vi "Create Webform.vi"(6 "Under Construction":bool[](array[boolean]), 8 "error in (no error)":errorcluster, 9 "Mathcad version":i32, 10 "Method Name":string, 11 "Method":T2) -> (0 "error out":errorcluster, 3 "HTML string":string)   [LabVIEW 2012, in "Design Server.lvlib"]
uses:
  Design Server.lvlib
  Method.ctl
  RequestKeys.ctl
  Folders.ctl
  <vilib>/Utility/file.llb/Read From Spreadsheet File (string).vi
panel:
  in  "Required":bool[](array[boolean])=[TRUE, TRUE, TRUE, TRUE, FALSE, FALSE, FALSE, FALSE]
  out "String":string
  in  "Load countries":bool
  in  "Country codes":string[][](array[string])=[["\"Table 1. Countries, Dependencies, and Areas of Special Sovereignty (Alphabetical by Name)\"", "", ""], ["http://earth-info.nga.mil/gns/html/gazetteers2.html", "", ""], ["Code", "Name (Upper Case)", "Name (Upper and Lower Case)"], ["AF", "AFGHANISTAN", "Afghanistan"], ["AX", "AKROTIRI", "Akrotiri"], ["AL", "ALBANIA", "Albania"], ["AG", "ALGERIA", "Algeria"], ["AQ", "AMERICAN SAMOA", "American Samoa"], ["AN", "ANDORRA", "Andorra"], ["AO", "ANGOLA", "Angola"], ["AV", "ANGUILLA", "Anguilla"], ["AY", "ANTARCTICA", "Antarctica"], ["AC", "ANTIGUA AND BARBUDA", "Antigua and Barbuda"], ["AR", "ARGENTINA", "Argentina"], ["AM", "ARMENIA", "Armenia"], ["AA", "ARUBA", "Aruba"], ["AT", "ASHMORE AND CARTIER ISLANDS", "Ashmore and Cartier Islands"], ["AS", "AUSTRALIA", "Australia"], ["AU", "AUSTRIA", "Austria"], ["AJ", "AZERBAIJAN", "Azerbaijan"], ["BF", "BAHAMAS, THE", "Bahamas, The"], ["BA", "BAHRAIN", "Bahrain"], ["FQ", "BAKER ISLAND", "Baker Island"], ["BG", "BANGLADESH", "Bangladesh"], ["BB", "BARBADOS", "Barbados"], ["BS", "BASSAS DA INDIA", "Bassas da India"], ["BO", "BELARUS", "Belarus"], ["BE", "BELGIUM", "Belgium"], ["BH", "BELIZE", "Belize"], ["BN", "BENIN", "Benin"], ["BD", "BERMUDA", "Bermuda"], ["BT", "BHUTAN", "Bhutan"], ["BL", "BOLIVIA", "Bolivia"], ["BK", "BOSNIA AND HERZEGOVINA", "Bosnia and Herzegovina"], ["BC", "BOTSWANA", "Botswana"], ["BV", "BOUVET ISLAND", "Bouvet Island"], ["BR", "BRAZIL", "Brazil"], ["IO", "BRITISH INDIAN OCEAN TERRITORY", "British Indian Ocean Territory"], ["BX", "BRUNEI", "Brunei"], ["BU", "BULGARIA", "Bulgaria"], ["UV", "BURKINA FASO", "Burkina Faso"], ["BM", "BURMA", "Burma"], ["BY", "BURUNDI", "Burundi"], ["CB", "CAMBODIA", "Cambodia"], ["CM", "CAMEROON", "Cameroon"], ["CA", "CANADA", "Canada"], ["CV", "CAPE VERDE", "Cape Verde"], ["CJ", "CAYMAN ISLANDS", "Cayman Islands"], ["CT", "CENTRAL AFRICAN REPUBLIC", "Central African Republic"], ["CD", "CHAD", "Chad"], ["CI", "CHILE", "Chile"], ["CH", "CHINA", "China"], ["KT", "CHRISTMAS ISLAND", "Christmas Island"], ["IP", "CLIPPERTON ISLAND", "Clipperton Island"], ["CK", "COCOS (KEELING) ISLANDS", "Cocos (Keeling) Islands"], ["CO", "COLOMBIA", "Colombia"], ["CN", "COMOROS", "Comoros"], ["CF", "CONGO (BRAZZAVILLE)", "Congo (Brazzaville)"], ["CG", "CONGO (KINSHASA)", "Congo (Kinshasa)"], ["CW", "COOK ISLANDS", "Cook Islands"], ["CR", "CORAL SEA ISLANDS", "Coral Sea Islands"], ["CS", "COSTA RICA", "Costa Rica"], ["IV", "CÔTE D’IVOIRE", "Côte d’Ivoire"], ["HR", "CROATIA", "Croatia"], ["CU", "CUBA", "Cuba"], ["UC", "CURAÇAO", "Curaçao"], ["CY", "CYPRUS", "Cyprus"], ["EZ", "CZECH REPUBLIC", "Czech Republic"], ["DA", "DENMARK", "Denmark"], ["DX", "DHEKELIA", "Dhekelia"], ["DJ", "DJIBOUTI", "Djibouti"], ["DO", "DOMINICA", "Dominica"], ["DR", "DOMINICAN REPUBLIC", "Dominican Republic"], ["EC", "ECUADOR", "Ecuador"], ["EG", "EGYPT", "Egypt"], ["ES", "EL SALVADOR", "El Salvador"], ["EK", "EQUATORIAL GUINEA", "Equatorial Guinea"], ["ER", "ERITREA", "Eritrea"], ["EN", "ESTONIA", "Estonia"], ["ET", "ETHIOPIA", "Ethiopia"], ["PJ", "ETOROFU, HABOMAI, KUNASHIRI, AND SHIKOTAN ISLANDS", "Etorofu, Habomai, Kunashiri, and Shikotan Islands"], ["EU", "EUROPA ISLAND", "Europa Island"], ["FK", "FALKLAND ISLANDS (ISLAS MALVINAS)", "Falkland Islands (Islas Malvinas)"], ["FO", "FAROE ISLANDS", "Faroe Islands"], ["FJ", "FIJI", "Fiji"], ["FI", "FINLAND", "Finland"], ["FR", "FRANCE", "France"], ["FG", "FRENCH GUIANA", "French Guiana"], ["FP", "FRENCH POLYNESIA", "French Polynesia"], ["FS", "FRENCH SOUTHERN AND ANTARCTIC LANDS", "French Southern and Antarctic Lands"], ["GB", "GABON", "Gabon"], ["GA", "GAMBIA, THE", "Gambia, The"], ["GZ", "GAZA STRIP", "Gaza Strip"], ["GG", "GEORGIA", "Georgia"], ["GM", "GERMANY", "Germany"], ["GH", "GHANA", "Ghana"], ["GI", "GIBRALTAR", "Gibraltar"], ["GO", "GLORIOSO ISLANDS", "Glorioso Islands"], ["GR", "GREECE", "Greece"], ["GL", "GREENLAND", "Greenland"], ["GJ", "GRENADA", "Grenada"], ["GP", "GUADELOUPE", "Guadeloupe"], ["GQ", "GUAM", "Guam"], ["GT", "GUATEMALA", "Guatemala"], ["GK", "GUERNSEY", "Guernsey"], ["GV", "GUINEA", "Guinea"], ["PU", "GUINEA-BISSAU", "Guinea-Bissau"], ["GY", "GUYANA", "Guyana"], ["HA", "HAITI", "Haiti"], ["HM", "HEARD ISLAND AND MCDONALD  ISLANDS", "Heard Island and McDonald  Islands"], ["HO", "HONDURAS", "Honduras"], ["HK", "HONG KONG", "Hong Kong"], ["HQ ", "HOWLAND ISLAND", "Howland Island"], ["HU", "HUNGARY", "Hungary"], ["IC", "ICELAND", "Iceland"], ["IN", "INDIA", "India"], ["ID", "INDONESIA", "Indonesia"], ["IR", "IRAN", "Iran"], ["IZ", "IRAQ", "Iraq"], ["EI", "IRELAND", "Ireland"], ["IM", "ISLE OF MAN", "Isle of Man"], ["IS", "ISRAEL", "Israel"], ["IT", "ITALY", "Italy"], ["JM", "JAMAICA", "Jamaica"], ["JN", "JAN MAYEN", "Jan Mayen"], ["JA", "JAPAN", "Japan"], ["DQ", "JARVIS ISLAND", "Jarvis Island"], ["JE", "JERSEY", "Jersey"], ["JQ", "JOHNSTON ATOLL", "Johnston Atoll"], ["JO", "JORDAN", "Jordan"], ["JU", "JUAN DE NOVA ISLAND", "Juan de Nova Island"], ["KZ", "KAZAKHSTAN", "Kazakhstan"], ["KE", "KENYA", "Kenya"], ["KQ", "KINGMAN REEF", "Kingman Reef"], ["KR", "KIRIBATI", "Kiribati"], ["KN", "KOREA, NORTH", "Korea, North"], ["KS", "KOREA, SOUTH", "Korea, South"], ["KV", "KOSOVO", "Kosovo"], ["KU", "KUWAIT", "Kuwait"], ["KG", "KYRGYZSTAN", "Kyrgyzstan"], ["LA", "LAOS", "Laos"], ["LG", "LATVIA", "Latvia"], ["LE", "LEBANON", "Lebanon"], ["LT", "LESOTHO", "Lesotho"], ["LI", "LIBERIA", "Liberia"], ["LY", "LIBYA", "Libya"], ["LS", "LIECHTENSTEIN", "Liechtenstein"], ["LH", "LITHUANIA", "Lithuania"], ["LU", "LUXEMBOURG", "Luxembourg"], ["MC", "MACAU", "Macau"], ["MK", "MACEDONIA", "Macedonia"], ["MA", "MADAGASCAR", "Madagascar"], ["MI", "MALAWI", "Malawi"], ["MY", "MALAYSIA", "Malaysia"], ["MV", "MALDIVES", "Maldives"], ["ML", "MALI", "Mali"], ["MT", "MALTA", "Malta"], ["RM", "MARSHALL ISLANDS", "Marshall Islands"], ["MB", "MARTINIQUE", "Martinique"], ["MR", "MAURITANIA", "Mauritania"], ["MP", "MAURITIUS", "Mauritius"], ["MF", "MAYOTTE", "Mayotte"], ["MX", "MEXICO", "Mexico"], ["FM", "MICRONESIA, FEDERATED STATES OF", "Micronesia, Federated States of"], ["MQ ", "MIDWAY ISLANDS", "Midway Islands"], ["MD", "MOLDOVA", "Moldova"], ["MN", "MONACO", "Monaco"], ["MG", "MONGOLIA", "Mongolia"], ["MJ", "MONTENEGRO", "Montenegro"], ["MH", "MONTSERRAT", "Montserrat"], ["MO", "MOROCCO", "Morocco"], ["MZ", "MOZAMBIQUE", "Mozambique"], ["WA", "NAMIBIA", "Namibia"], ["NR", "NAURU", "Nauru"], ["BQ", "NAVASSA ISLAND", "Navassa Island"], ["NP", "NEPAL", "Nepal"], ["NL", "NETHERLANDS", "Netherlands"], ["NC", "NEW CALEDONIA", "New Caledonia"], ["NZ", "NEW ZEALAND", "New Zealand"], ["NU", "NICARAGUA", "Nicaragua"], ["NG", "NIGER", "Niger"], ["NI", "NIGERIA", "Nigeria"], ["NE", "NIUE", "Niue"], ["NF", "NORFOLK ISLAND", "Norfolk Island"], ["CQ", "NORTHERN MARIANA ISLANDS", "Northern Mariana Islands"], ["NO", "NORWAY", "Norway"], ["MU", "OMAN", "Oman"], ["PK", "PAKISTAN", "Pakistan"], ["PS", "PALAU", "Palau"], ["LQ", "PALMYRA ATOLL", "Palmyra Atoll"], ["PM", "PANAMA", "Panama"], ["PP", "PAPUA NEW GUINEA", "Papua New Guinea"], ["PF", "PARACEL ISLANDS", "Paracel Islands"], ["PA", "PARAGUAY", "Paraguay"], ["PE", "PERU", "Peru"], ["RP", "PHILIPPINES", "Philippines"], ["PC", "PITCAIRN ISLANDS", "Pitcairn Islands"], ["PL", "POLAND", "Poland"], ["PO", "PORTUGAL", "Portugal"], ["RQ", "PUERTO RICO", "Puerto Rico"], ["QA", "QATAR", "Qatar"], ["RE", "REUNION", "Reunion"], ["RO", "ROMANIA", "Romania"], ["RS", "RUSSIA", "Russia"], ["RW", "RWANDA", "Rwanda"], ["TB", "SAINT BARTHELEMY", "Saint Barthelemy"], ["SH", "SAINT HELENA, ASCENSION, AND TRISTAN DA CUNHA", "Saint Helena, Ascension, and Tristan da Cunha"], ["SC", "SAINT KITTS AND NEVIS", "Saint Kitts and Nevis"], ["ST", "SAINT LUCIA", "Saint Lucia"], ["RN", "SAINT MARTIN", "Saint Martin"], ["SB", "SAINT PIERRE AND MIQUELON", "Saint Pierre and Miquelon"], ["VC", "SAINT VINCENT AND THE GRENADINES", "Saint Vincent and the Grenadines"], ["WS", "SAMOA", "Samoa"], ["SM", "SAN MARINO", "San Marino"], ["TP", "SAO TOME AND PRINCIPE", "Sao Tome and Principe"], ["SA", "SAUDI ARABIA", "Saudi Arabia"], ["SG", "SENEGAL", "Senegal"], ["RI", "SERBIA", "Serbia"], ["SE", "SEYCHELLES", "Seychelles"], ["SL", "SIERRA LEONE", "Sierra Leone"], ["SN", "SINGAPORE", "Singapore"], ["NN", "SINT MAARTEN", "Sint Maarten"], ["LO", "SLOVAKIA", "Slovakia"], ["SI", "SLOVENIA", "Slovenia"], ["BP", "SOLOMON ISLANDS", "Solomon Islands"], ["SO", "SOMALIA", "Somalia"], ["SF", "SOUTH AFRICA", "South Africa"], ["SX", "SOUTH GEORGIA AND SOUTH SANDWICH ISLANDS", "South Georgia and South Sandwich Islands"], ["OD", "SOUTH SUDAN", "South Sudan"], ["SP", "SPAIN", "Spain"], ["PG", "SPRATLY ISLANDS", "Spratly Islands"], ["CE", "SRI LANKA", "Sri Lanka"], ["SU", "SUDAN", "Sudan"], ["NS", "SURINAME", "Suriname"], ["SV", "SVALBARD", "Svalbard"], ["WZ", "SWAZILAND", "Swaziland"], ["SW", "SWEDEN", "Sweden"], ["SZ", "SWITZERLAND", "Switzerland"], ["SY", "SYRIA", "Syria"], ["TW", "TAIWAN", "Taiwan"], ["TI", "TAJIKISTAN", "Tajikistan"], ["TZ", "TANZANIA", "Tanzania"], ["TH", "THAILAND", "Thailand"], ["TT", "TIMOR-LESTE", "Timor-Leste"], ["TO", "TOGO", "Togo"], ["TL", "TOKELAU", "Tokelau"], ["TN", "TONGA", "Tonga"], ["TD", "TRINIDAD AND TOBAGO", "Trinidad and Tobago"], ["TE", "TROMELIN ISLAND", "Tromelin Island"], ["TS", "TUNISIA", "Tunisia"], ["TU", "TURKEY", "Turkey"], ["TX", "TURKMENISTAN", "Turkmenistan"], ["TK", "TURKS AND CAICOS ISLANDS", "Turks and Caicos Islands"], ["TV", "TUVALU", "Tuvalu"], ["UG", "UGANDA", "Uganda"], ["UP", "UKRAINE", "Ukraine"], ["AE", "UNITED ARAB EMIRATES", "United Arab Emirates"], ["UK", "UNITED KINGDOM", "United Kingdom"], ["US", "UNITED STATES", "United States"], ["UY", "URUGUAY", "Uruguay"], ["UZ", "UZBEKISTAN", "Uzbekistan"], ["NH", "VANUATU", "Vanuatu"], ["VT", "VATICAN CITY", "Vatican City"], ["VE", "VENEZUELA", "Venezuela"], ["VM", "VIETNAM", "Vietnam"], ["VI", "VIRGIN ISLANDS, BRITISH", "Virgin Islands, British"], ["VQ ", "VIRGIN ISLANDS, U.S.", "Virgin Islands, U.S."], ["WQ", "WAKE ISLAND", "Wake Island"], ["WF", "WALLIS AND FUTUNA", "Wallis and Futuna"], ["WE", "WEST BANK", "West Bank"], ["WI", "WESTERN SAHARA", "Western Sahara"], ["YM", "YEMEN", "Yemen"], ["ZA", "ZAMBIA", "Zambia"], ["ZI", "ZIMBABWE", "Zimbabwe"]]
  in  "Path":path=path "C:/Users/design/Documents/LabVIEW Code/AguaClara Design Server/Country codes.txt"
  in  "Request Keys":T1=enum."ProjectNotes"
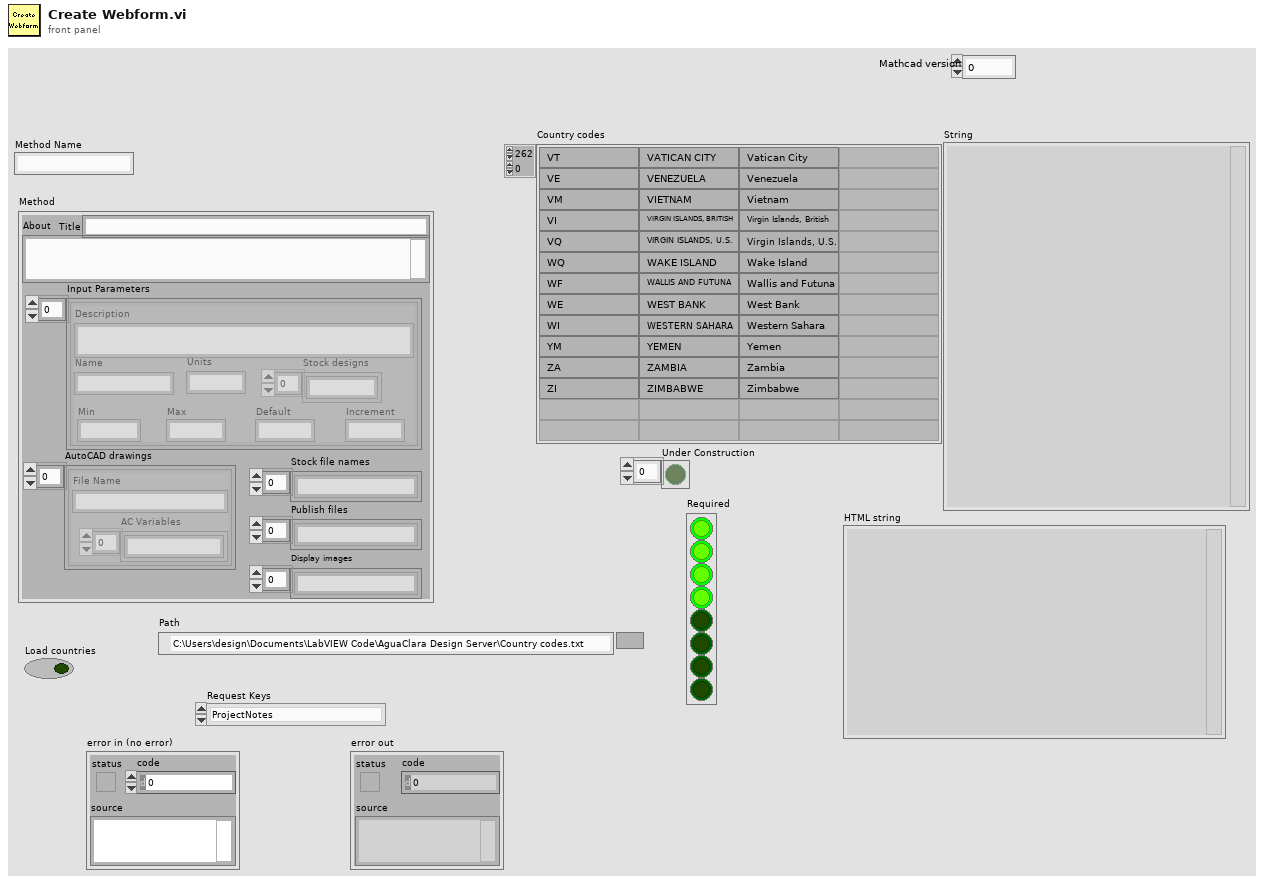
[diagram p1: front panel]
types:
  T1 = typedef "Design Server.lvlib/RequestKeys.ctl" = enum16{"FormName", "Name", "Email", "Organization", "Country", "ProjectTitle", "ProjectCity", "ProjectState", "ProjectNotes"}
  T2 = typedef "Method.ctl" = cluster{"Title":string, "About":string, "Input Parameters":cluster{"Description":string, "Name":string, "Min":string, "Max":string, "Default":string, "Units":string, "Increment":string, "Stock designs":string[]}[], "AutoCAD drawings":cluster{"File Name":string, "AC Variables":string[]}[], "Stock file names":string[], "Publish files":string[], "Display images":string[]}
  T3 = typedef "Design Server.lvlib/Folders.ctl" = enum16{"MathcadMethods", "RequestedDesigns", "CompletedDesigns", "MathcadCode", "CollabnetSVN.exe"}
  T4 = enum16{"open", "replace", "create", "open or create", "replace or create", "replace or create with confirmation"}
  T5 = cluster{"Description":string, "Name":string, "Min":string, "Max":string, "Default":string, "Units":string, "Increment":string, "Stock designs":string[]}[]
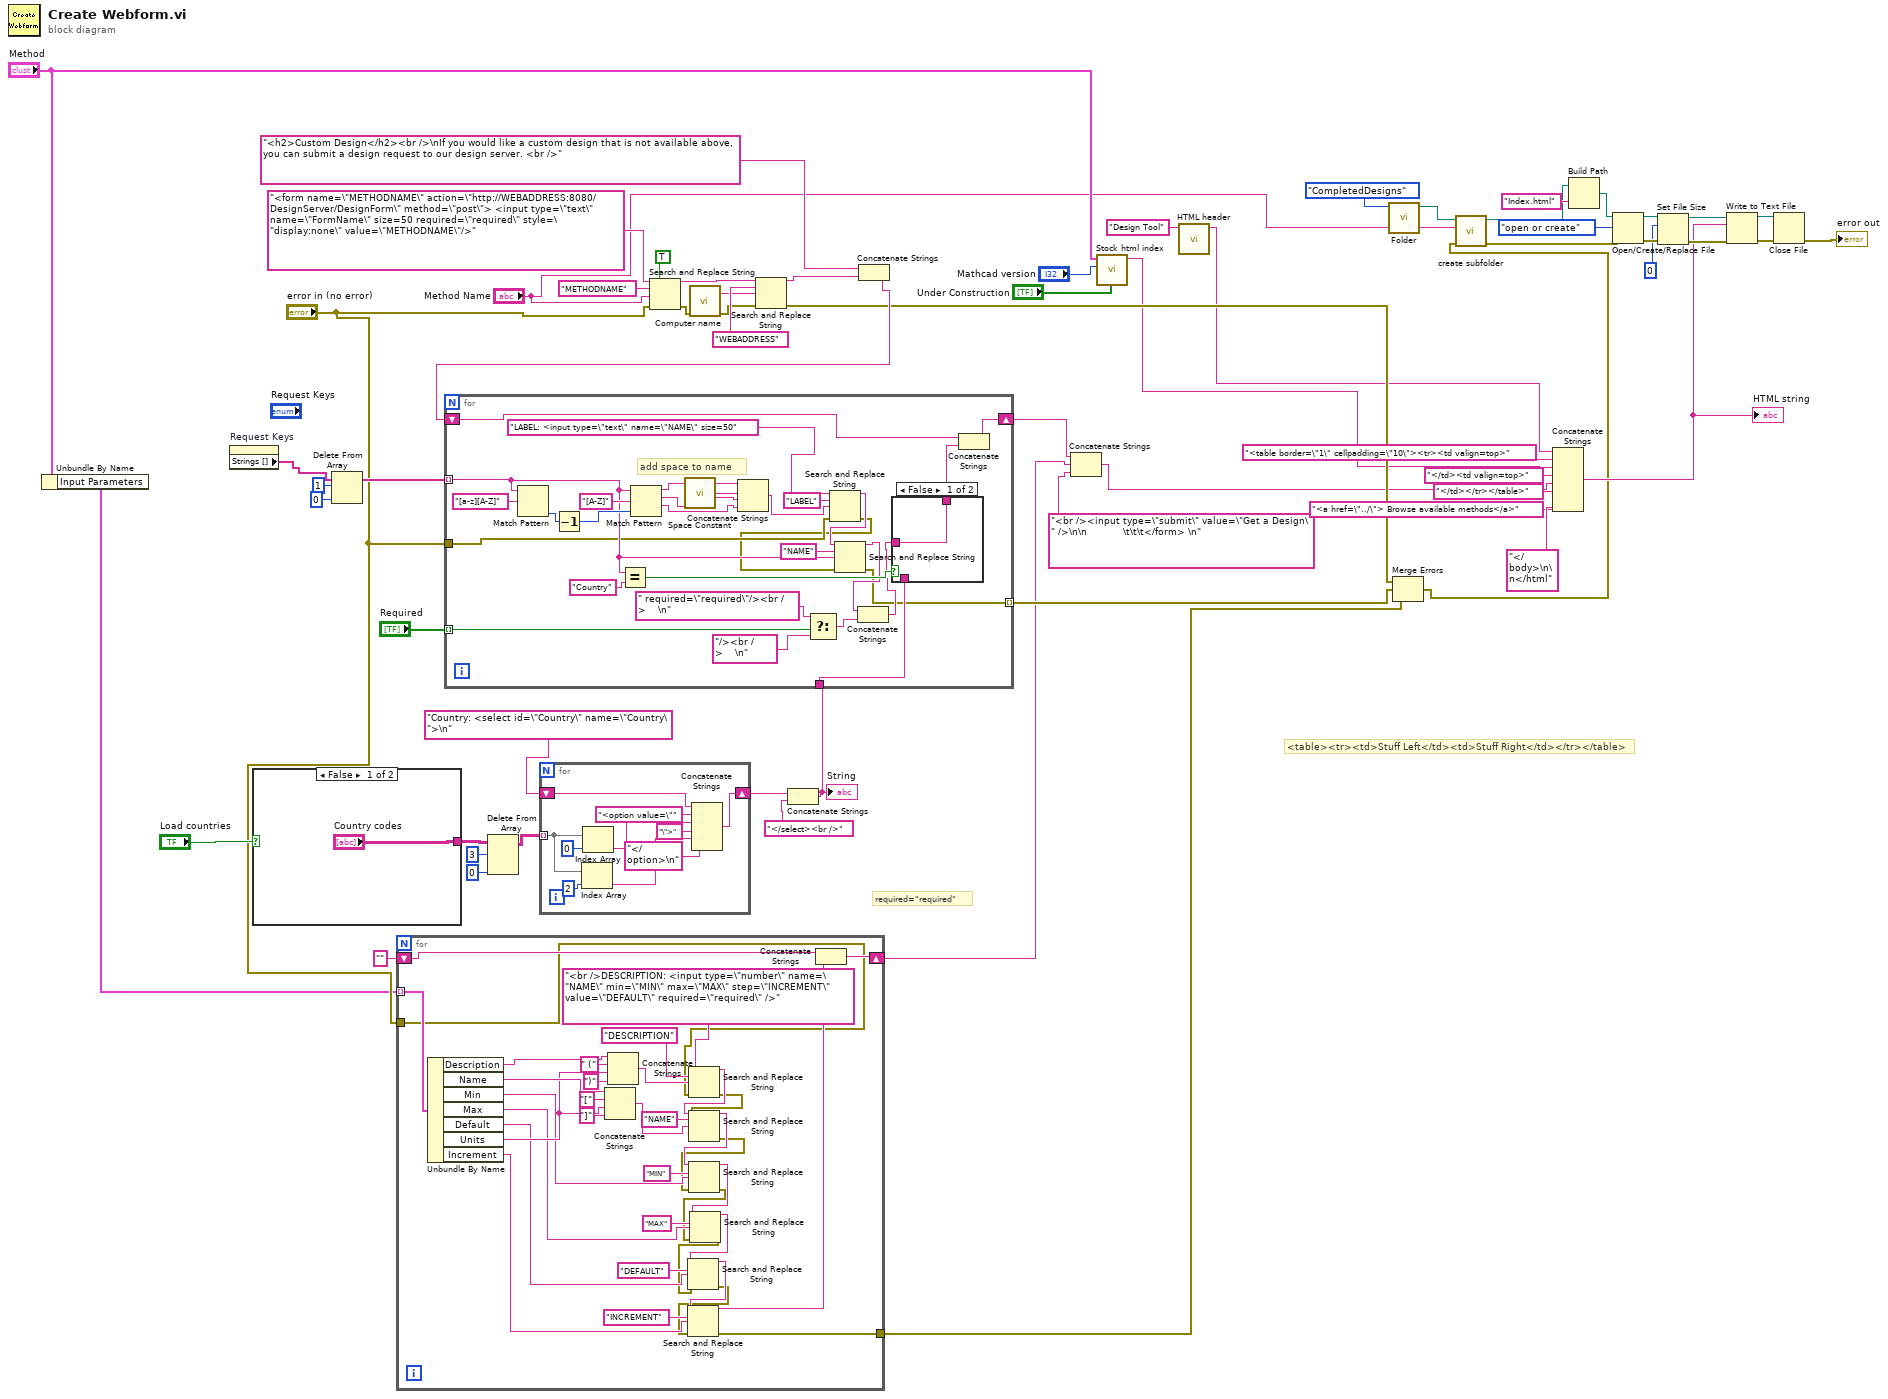
[diagram p0: block diagram]
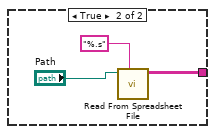
[diagram p3: hidden frame]
diagram:
  # "<table><tr><td>Stuff Left</td><td>Stuff Right</td></tr></table>"
  # "required=\"required\""
  n1 = Unbundle By Name("Method") -> ("Input Parameters"=w34:T5)
  n2 = property on="Request Keys" class="Enum (strict)"() -> ("Strings []"=w54:string[])  [unwired: 2 in, 2 out]
  n3 = case shown="False" "Load countries" {
    tunnel: ["Country codes" w66] -> w61
    frame False {
    }
    frame True {
      n4 = call-poly <vilib>:"Read From Spreadsheet File.vi"("format (%s)"="%.s" ("format (%.3f)"), "file path (dialog if empty)"="Path") -> ("all rows"=w66:string[][])  [unwired: 5 in, 4 out]
    }
  }
  n5 = Delete From Array(array=w54, length=1, index=0) -> (array with subset deleted=w51:string[])  [unwired: 1 out]
  n6 = for {
    tunnel: w34 -> [w104] mode=indexing
    shift-right: [w79] -> w10
    shift-left: "" -> [w80]
    tunnel: "error in (no error)" -> [w75]
    tunnel: [w69] -> w37
    n7 = Unbundle By Name(w104) -> ("Description"=w78:string, "Name"=w98:string, "Min"=w88:string, "Max"=w87:string, "Default"=w86:string, "Units"=w96:string, "Increment"=w85:string)
    n8 = Concatenate Strings(w98, "[" ("string"), w96, "]" ("string")) -> (w94:string)
    n9 = Concatenate Strings(w78, " (" ("string"), w96, ")" ("string")) -> (w101:string)
    n10 = Search and Replace String(input string="<br />DESCRIPTION: <input type=\"number\" name=\"NAME\" min=\"MIN\" max=\"MAX\" step=\"INCREMENT\" value=\"DEFAULT\" required=\"required\" />", search string="DESCRIPTION", replace string=w101, error in=w75) -> (result string=w100:string, error out=w74:errorcluster)  [unwired: 4 in, 2 out]
    n11 = Search and Replace String(input string=w100, search string="NAME", replace string=w94, error in=w74) -> (result string=w93:string, error out=w73:errorcluster)  [unwired: 4 in, 2 out]
    n12 = Search and Replace String(input string=w93, search string="MIN", replace string=w88, error in=w73) -> (result string=w84:string, error out=w72:errorcluster)  [unwired: 4 in, 2 out]
    n13 = Search and Replace String(input string=w84, search string="MAX", replace string=w87, error in=w72) -> (result string=w83:string, error out=w71:errorcluster)  [unwired: 4 in, 2 out]
    n14 = Search and Replace String(input string=w83, search string="DEFAULT", replace string=w86, error in=w71) -> (result string=w82:string, error out=w70:errorcluster)  [unwired: 4 in, 2 out]
    n15 = Search and Replace String(input string=w82, search string="INCREMENT", replace string=w85, error in=w70) -> (result string=w81:string, error out=w69:errorcluster)  [unwired: 4 in, 2 out]
    n16 = Concatenate Strings(w80, w81) -> (w79:string)
  }
  n17 = Delete From Array(array=w61, length=3, index (row)=0) -> (array with subset deleted=w60:string[][])  [unwired: 1 in, 1 out]
  n18 = for {
    tunnel: w60 -> [w112] mode=indexing
    shift-right: [w105] -> w56
    shift-left: "Country: <select id=\"Country\" name=\"Country\">\n" -> [w106]
    n19 = Index Array(array=w112, index=2) -> (element=w108:string)
    n20 = Index Array(array=w112, index=0) -> (element=w110:string)
    n21 = Concatenate Strings(w106, "<option value=\"" ("string"), w110, "\">" ("string"), w108, "</option>\n" ("string")) -> (w105:string)
  }
  n22 = Search and Replace String(replace all?=TRUE ("replace all? (F)"), input string="<form name=\"METHODNAME\" action=\"http://WEBADDRESS:8080/DesignServer/DesignForm\" method=\"post\"> <input type=\"text\" name=\"FormName\" size=50 required=\"required\" style=\"display:none\" value=\"METHODNAME\"/>", search string="METHODNAME", replace string="Method Name", error in="error in (no error)") -> (result string=w45:string, error out=w41:errorcluster)  [unwired: 3 in, 2 out]
  n23 = call "Computer name.vi"("error in (no error)"=w41) -> ("error out"=w40:errorcluster, "Computer web address"=w42:string)  [unwired: 8 in, 1 out]
  n24 = Search and Replace String(input string=w45, search string="WEBADDRESS", replace string=w42, error in=w40) -> (result string=w43:string, error out=w20:errorcluster)  [unwired: 4 in, 2 out]
  n25 = Concatenate Strings(w56, "</select><br />") -> (w50:string)
  "String" <- w50
  n26 = Concatenate Strings("<h2>Custom Design</h2><br />\nIf you would like a custom design that is not available above, you can submit a design request to our design server. <br />", w43) -> (w46:string)
  n27 = for {
    tunnel: w51 -> [w127] mode=indexing
    shift-right: [w129] -> w11
    shift-left: w46 -> [w130]
    tunnel: w50 -> [w125]
    tunnel: "Required" -> [w121] mode=indexing
    tunnel: "error in (no error)" -> [w117]
    tunnel: [w115] -> w39 mode=indexing
    # "add space to name"
    n28 = Match Pattern(string=w127, regular expression="[a-z][A-Z]") -> (offset past match=w142:i32)  [unwired: 1 in, 3 out]
    n29 = Decrement(x=w142) -> (x-1=w141:i32)
    n30 = Equal?(x=w127, y="Country") -> (x = y?=w126:bool)
    n31 = Match Pattern(string=w127, regular expression="[A-Z]", offset (0)=w141) -> (before substring=w139:string, match substring=w137:string, after substring=w136:string)  [unwired: 1 out]
    n32 = call <vilib>:"Space Constant.vi"() -> ("String"=w138:string)
    n33 = Concatenate Strings(w139, w138, w137, w136) -> (w133:string)
    n34 = Select(t=" required=\"required\"/><br />    \n", s=w121, f="/><br />    \n") -> (s? t:f=w119:string)
    n35 = Search and Replace String(input string="LABEL: <input type=\"text\" name=\"NAME\" size=50", search string="LABEL", replace string=w133, error in=w117) -> (result string=w132:string, error out=w116:errorcluster)  [unwired: 4 in, 2 out]
    n36 = Search and Replace String(input string=w132, search string="NAME", replace string=w127, error in=w116) -> (result string=w123:string, error out=w115:errorcluster)  [unwired: 4 in, 2 out]
    n37 = Concatenate Strings(w123, w119) -> (w118:string)
    n38 = case shown="False" w126 {
      tunnel: w118 -> [w144 _]
      tunnel: w125 -> [_ w145]
      tunnel: [w144 w145] -> w124
      frame False {
      }
      frame True {
      }
    }
    n39 = Concatenate Strings(w130, w124) -> (w129:string)
  }
  n40 = Concatenate Strings(w11, w10, "<br /><input type=\"submit\" value=\"Get a Design\" />\n\n            \t\t\t</form> \n" ("string")) -> (w8:string)
  n41 = call "Stock html index.vi"("Under Construction"="Under Construction", "Mathcad version"="Mathcad version", "Method"="Method") -> ("HTML"=w13:string)  [unwired: 8 in]
  n42 = call "HTML header.vi"("Title"="Design Tool") -> ("HTML header"=w15:string)  [unwired: 10 in]
  n43 = call "Folder.vi"("Folders"=Folders."CompletedDesigns") -> ("FolderPath"=w22:path)  [unwired: 8 in, 2 out]
  n44 = Merge Errors(w20, w39, w37) -> (w1:errorcluster)
  n45 = call "create subfolder.vi"("error in (no error)"=w1, "Folder Name"="Method Name", "FolderPath"=w22) -> ("error out"=w2:errorcluster, "Subfolder path"=w3:path)  [unwired: 7 in]
  n46 = Concatenate Strings(w15, "<table border=\"1\" cellpadding=\"10\"><tr><td valign=top>" ("string"), w13, "</td><td valign=top>" ("string"), w8, "</td></tr></table>" ("string"), "<a href=\"../\"> Browse available methods</a>" ("string"), "</body>\n\n</html") -> (w6:string)
  "HTML string" <- w6
  n47 = Build Path(base path=w3, name or relative path="Index.html") -> (appended path=w31:path)
  n48 = Open/Create/Replace File(file path (use dialog)=w31, error in=w2, operation (0:open)=T4."open or create") -> (refnum out=w28:refnum<file>, error out=w26:errorcluster)  [unwired: 3 in, 1 out]
  n49 = Set File Size(4:w26, 6:i64 0 ("size (in bytes)"), 7:w28) -> (0:w25:errorcluster, 3:w27:refnum<file>)
  n50 = Write to Text File(file (use dialog)=w27, text=w6, error in=w25) -> (refnum out=w29:refnum<file>, error out=w30:errorcluster)  [unwired: 1 in, 1 out]
  n51 = Close File(refnum=w29, error in=w30) -> (error out=→"error out":errorcluster)  [unwired: 1 out]
